vi "frequency report.vi"(8 "Pattern frequency (Hz)":dbl, 9 "Frecuencias validas":bool[](array[boolean]), 10 "Magnitud*df":dbl[](array[numeric])) -> (1 "continuar?":bool, 3 "Report":string)   [LabVIEW 2015]
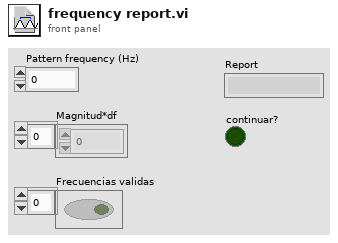
[diagram p1: front panel]
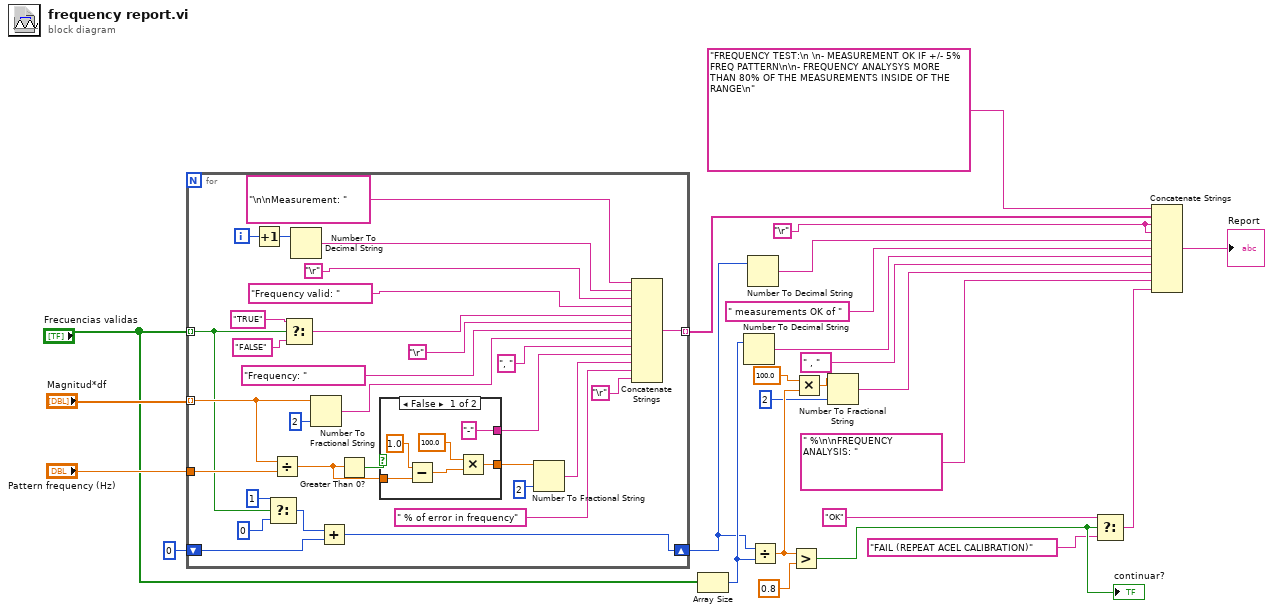
[diagram p0: block diagram]
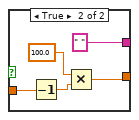
[diagram p2: hidden frame]
diagram:
  w18 = "\r"
  n1 = for {
    tunnel: "Frecuencias validas" -> [w34] mode=indexing
    tunnel: "Magnitud*df" -> [w53] mode=indexing
    tunnel: "Pattern frequency (Hz)" -> [w52]
    tunnel: [w35] -> w3 mode=indexing
    shift-right: [w29] -> w5
    shift-left: 0 -> [w30]
    i -> [w55]
    n2 = Increment(x=w55) -> (x+1=w54:i32)
    n3 = Select(t=1, s=w34, f=0) -> (s? t:f=w31:i32)
    n4 = Divide(x=w53, y=w52) -> (x/y=w50:dbl)
    n5 = Select(t="TRUE", s=w34, f="FALSE") -> (s? t:f=w44:string)
    n6 = Number To Decimal String(number=w54) -> (decimal integer string=w47:string)  [unwired: 1 in]
    n7 = Number To Fractional String(number=w53, precision (6)=i16 2) -> (F-format string=w41:string)  [unwired: 2 in]
    n8 = Add(x=w31, y=w30) -> (x+y=w29:i32)
    n9 = Greater Than 0?(x=w50) -> (x > 0?=w51:bool)
    n10 = case shown="False" w51 {
      tunnel: w50 -> [w62 w64]
      tunnel: [w59 w66] -> w49
      tunnel: ["-" " "] -> w39
      frame False {
        n11 = Subtract(x=1.0, y=w62) -> (x-y=w57:dbl)
        n12 = Multiply(x=100.0, y=w57) -> (x*y=w59:dbl)
      }
      frame True {
        n13 = Decrement(x=w64) -> (x-1=w65:dbl)
        n14 = Multiply(x=100.0, y=w65) -> (x*y=w66:dbl)
      }
    }
    n15 = Number To Fractional String(number=w49, precision (6)=i16 2) -> (F-format string=w38:string)  [unwired: 2 in]
    n16 = Concatenate Strings("\n\nMeasurement: ", w47, "\r", "Frequency valid: ", w44, "\r", "Frequency: ", w41, ", ", w39, w38, " % of error in frequency", "\r") -> (w35:string)
  }
  n17 = Array Size(array="Frecuencias validas") -> (size(s)=w6:i32)
  n18 = Number To Decimal String(number=w6) -> (decimal integer string=w11:string)  [unwired: 1 in]
  n19 = Number To Decimal String(number=w5) -> (decimal integer string=w17:string)  [unwired: 1 in]
  n20 = Divide(x=w5, y=w6) -> (x/y=w20:dbl)
  n21 = Greater?(x=w20, y=0.8) -> (0:w15:bool)
  "continuar?" <- w15
  n22 = Multiply(x=100.0, y=w20) -> (x*y=w21:dbl)
  n23 = Number To Fractional String(number=w21, precision (6)=i16 2) -> (F-format string=w12:string)  [unwired: 2 in]
  n24 = Select(t="OK", s=w15, f="FAIL (REPEAT ACEL CALIBRATION)") -> (s? t:f=w14:string)
  n25 = Concatenate Strings("FREQUENCY TEST:\n \n- MEASUREMENT OK IF +/- 5% FREQ PATTERN\n\n- FREQUENCY ANALYSYS MORE THAN 80% OF THE MEASUREMENTS INSIDE OF THE RANGE\n", w3, w18, w18, w17, " measurements OK of ", w11, " , ", w12, " %\n\nFREQUENCY ANALYSIS: ", w14) -> (→"Report":string)
